vi "Open Motors.vi"() -> ()   [LabVIEW 2018]
uses:
  <vilib>/Rock Robotics/WPI/ThirdParty/Phoenix-LabVIEW/Motor Controller/Controls/CTRE_Phoenix_MotorControl_StatusFrameEnhanced.ctl
  <vilib>/Rock Robotics/WPI/ThirdParty/Phoenix-LabVIEW/Motor Controller/Controls/CTRE_Phoenix_MotorControl_EnhancedMotorControllerConfigurables.ctl
  <vilib>/Rock Robotics/WPI/ThirdParty/Phoenix-LabVIEW/Motor Controller/Controls/CTRE_Phoenix_MotorControl_BaseConfigurables.ctl
  <vilib>/Rock Robotics/WPI/ThirdParty/Phoenix-LabVIEW/Motor Controller/Controls/CTRE_Phoenix_MotorControl_VelocityMeasurementPeriod.ctl
  <vilib>/Rock Robotics/WPI/ThirdParty/Phoenix-LabVIEW/Motor Controller/Controls/CTRE_Phoenix_MotorControl_SlotStructure.ctl
  <vilib>/Rock Robotics/WPI/ThirdParty/Phoenix-LabVIEW/Motor Controller/Controls/CTRE_Phoenix_MotorControl_FilterStruct.ctl
  <vilib>/Rock Robotics/WPI/ThirdParty/Phoenix-LabVIEW/Motor Controller/Controls/CTRE_Phoenix_MotorControl_RemoteSourceType.ctl
  <vilib>/Rock Robotics/WPI/ThirdParty/Phoenix-LabVIEW/Controls/CTRE_Phoenix_CustomParamConfiguration.ctl
  <vilib>/Rock Robotics/WPI/ThirdParty/Phoenix-LabVIEW/Motor Controller/Controls/CTRE_Phoenix_MotorControl_FeedbackDevice.ctl
  <vilib>/Rock Robotics/WPI/ThirdParty/Phoenix-LabVIEW/Motor Controller/Controls/CTRE_Phoenix_MotorControl_SensorTermFeedbackDevice_Enhanced.ctl
  <vilib>/Rock Robotics/WPI/ThirdParty/Phoenix-LabVIEW/Motor Controller/Controls/CTRE_Phoenix_MotorControl_LimitSwitchNormal.ctl
  <vilib>/Rock Robotics/WPI/ThirdParty/Phoenix-LabVIEW/Motor Controller/Controls/CTRE_Phoenix_MotorControl_LimitSwitchSource_Local.ctl
  Robot Global Data.vi
  <vilib>/Rock Robotics/WPI/RobotDrive/WPI_RobotDriveOpen4MotorWithExistingMotors.vi
  <vilib>/Rock Robotics/WPI/ThirdParty/Phoenix-LabVIEW/Motor Controller/Controls/CTRE_Phoenix_MotorControl_ControlMode.ctl
  <vilib>/Rock Robotics/WPI/ThirdParty/Phoenix-LabVIEW/Motor Controller/Controls/CTRE_Phoenix_MotorControl_MotionProfileTrajectoryPoint.ctl
  <vilib>/Rock Robotics/WPI/ThirdParty/Phoenix-LabVIEW/Motor Controller/Closed Loop/Motion Profile/CTRE_Phoenix_MotorControl_BufferedTrajectoryPointStream_WriteAll.vi
panel:
  in  "Tune PIDF Manually?":bool
  in  "Front PIDF Values":cluster{"P":dbl, "I":dbl, "D":dbl, "F":dbl}
  in  "Back PIDF Values":cluster{"P":dbl, "I":dbl, "D":dbl, "F":dbl}
  out "Array":dbl[][](array[numeric])
  # "AFTER YOU HAVE THE \nGAINS YOU WANT, \nR-CLICK > DATA \nOPERATIONS > MAKE\nTHE CURRENT VALUE\nDEFAULT\n\nor just hard-code them"
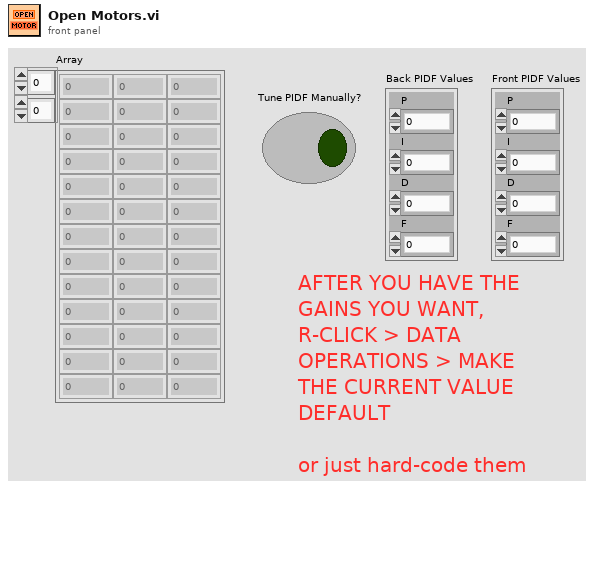
[diagram p1: front panel]
types:
  T1 = typedef "CTRE_Phoenix_MotorControl_EnhancedMotorControllerConfigurables.ctl" = cluster{"Base Configurables":T2, "primaryPID":cluster{"selectedFeedbackCoefficient":dbl, "selectedFeedbackSensor":T8}, "auxiliaryPID":cluster{"selectedFeedbackCoefficient":dbl, "selectedFeedbackSensor":T8}, "sum0Term":T9, "sum1Term":T9, "diff0Term":T9, "diff1Term":T9, "forwardLimitSwitchNormal":T10, "reverseLimitSwitchNormal":T10, "forwardLimitSwitchDeviceID":i32, "reverseLimitSwitchDeviceID":i32, "forwardLimitSwitchSource":T11, "reverseLimitSwitchSource":T11, "peakCurrentLimit":i32, "peakCurrentDuration":i32, "continuousCurrentLimit":i32}
  T2 = typedef "CTRE_Phoenix_MotorControl_BaseConfigurables.ctl" = cluster{"openLoopRamp":dbl, "closedLoopRamp":dbl, "peakOutputForward":dbl, "peakOutputReverse":dbl, "nominalOutputForward":dbl, "nominalOutputReverse":dbl, "neutralDeadband":dbl, "voltageCompSaturation":dbl, "voltageMeasurementFilter":i32, "velocityMeasurementPeriod":T3, "velocityMeasurementWindow":i32, "forwardSoftLimitThreshold":i32, "reverseSoftLimitThreshold":i32, "forwardSoftLimitEnable":bool, "reverseSoftLimitEnable":bool, "slot0":T4, "slot1":T4, "slot2":T4, "slot3":T4, "auxPIDPolarity":bool, "remoteFilter0":T5, "remoteFilter1":T5, "motionCruiseVelocity":i32, "motionAcceleration":i32, "motionProfileTrajectoryPeriod":i32, "feedbackNotContinuous":bool, "remoteSensorClosedLoopDisableNeutralOnLOS":bool, "clearPositionOnLimitF":bool, "clearPositionOnLimitR":bool, "clearPositionOnQuadIdx":bool, "limitSwitchDisableNeutralOnLOS":bool, "softLimitDisableNeutralOnLOS":bool, "pulseWidthPeriod_EdgesPerRot":i32, "pulseWidthPeriod_FilterWindowSz":i32, "customParam":T7, "trajectoryInterpolationEnable":bool}
  T3 = typedef "CTRE_Phoenix_MotorControl_VelocityMeasurementPeriod.ctl" = u16
  T4 = typedef "CTRE_Phoenix_MotorControl_SlotStructure.ctl" = cluster{"P":dbl, "I":dbl, "D":dbl, "F":dbl, "integralZone":dbl, "allowableClosedLoopError":i32, "maxIntegralAccumulator":dbl, "closedLoopPeakOutput":dbl, "closedLoopPeriod":i32}
  T5 = typedef "CTRE_Phoenix_MotorControl_FilterStruct.ctl" = cluster{"remoteSensorDeviceID":u8, "remoteSensorSource":T6}
  T6 = typedef "CTRE_Phoenix_MotorControl_RemoteSourceType.ctl" = enum16{"Off", "Talon SRX Selected Sensor", "Pigeon IMU Yaw", "Pigeon IMU Pitch", "Pigeon IMU Roll", "CANifier Quadrature", "CANifier PWM Input 0", "CANifier PWM Input 1", "CANifier PWM Input 2", "CANifier PWM Input 3", "Gadgeteer Pigeon Yaw", "Gadgeteer Pigeon Pitch", "Gadgeteer Pigeon Roll"}
  T7 = typedef "CTRE_Phoenix_CustomParamConfiguration.ctl" = cluster{"customParam0":i32, "customParam1":i32}
  T8 = typedef "CTRE_Phoenix_MotorControl_FeedbackDevice.ctl" = i8
  T9 = typedef "CTRE_Phoenix_MotorControl_SensorTermFeedbackDevice_Enhanced.ctl" = i8
  T10 = typedef "CTRE_Phoenix_MotorControl_LimitSwitchNormal.ctl" = enum16{"Normally Open", "Normally Closed", "Disabled"}
  T11 = typedef "CTRE_Phoenix_MotorControl_LimitSwitchSource_Local.ctl" = enum16{"Feedback Connector", "Remote Talon SRX", "Remote CANifier", "Deactivated"}
  T12 = typedef "CTRE_Phoenix_MotorControl_StatusFrameEnhanced.ctl" = u16
  T13 = typedef "CTRE_Phoenix_MotorControl_MotionProfileTrajectoryPoint.ctl" = cluster{"Position":dbl, "Velocity":dbl, "Arbitrary Feed Forward":dbl, "Auxiliary Position":dbl, "Auxiliary Velocity":dbl, "Auxiliary Arbitrary Feed Forward":dbl, "Profile Slot Select":i32, "Auxiliary Profile Slot Select":i32, "isLastPoint?":bool, "Zero Position?":bool, "durationMs":u32, "Use Aux PID?":bool}
  T14 = typedef "CTRE_Phoenix_MotorControl_BufferedTrajectoryPointStream_DeviceRef.ctl" = cluster{"Handle":u64, "Library Path":path}
  T15 = typedef "WPI_MotorControlDeviceRef.ctl" = cluster{"DeviceStatus":errorcluster, "Type":T16, "PWM":cluster{"PWM Channel":T17, "DeadBand":T18}, "CAN":cluster{"Device Number":u8, "SetOutput VI Ref":variant, "GetOutput VI Ref":variant, "Enable VI Ref":variant, "Disable VI Ref":variant, "Data":variant}, "Invert":bool, "DIO PWM":cluster{"PWM \"Enable\" Channel":T17, "DIOChannel":T19, "PWM Rate":dbl}}
  T16 = typedef "WPI_MotorControlType.ctl" = enum16{"PWM", "CAN", "DIO PWM"}
  T17 = typedef "FPGA_DIOPWMChannel.ctl" = enum8{"PWM 0", "PWM 1", "PWM 2", "PWM 3", "PWM 4", "PWM 5", "PWM 6", "PWM 7", "PWM 8", "PWM 9", "PWM MXP 0", "PWM MXP 1", "PWM MXP 2", "PWM MXP 3", "PWM MXP 4", "PWM MXP 5", "PWM MXP 6", "PWM MXP 7", "PWM MXP 8", "PWM MXP 9", "Invalid"}
  T18 = typedef "WPI_PWMDeadband.ctl" = cluster{"Name":string, "maxPositivePwm":i32, "minPositivePwm":i32, "centerPwm":i32, "maxNegativePwm":i32, "minNegativePwm":i32, "angularRange":u16}
  T19 = typedef "FPGA_DIOChannel.ctl" = enum8{"DIO 0", "DIO 1", "DIO 2", "DIO 3", "DIO 4", "DIO 5", "DIO 6", "DIO 7", "DIO 8", "DIO 9", "DIO MXP 0", "DIO MXP 1", "DIO MXP 2", "DIO MXP 3", "DIO MXP 4", "DIO MXP 5", "DIO MXP 6", "DIO MXP 7", "DIO MXP 8", "DIO MXP 9", "DIO MXP 10", "DIO MXP 11", "DIO MXP 12", "DIO MXP 13", "DIO MXP 14", "DIO MXP 15", "SPI Port CS1", "SPI Port CS2", "SPI Port CS3", "SPI Port MISO", "SPI Port MOSI", "Invalid"}
  T20 = typedef "Which Robot Enum.ctl" = enum16{"Competition Bot", "Practice Bot", "Code Bot"}
  T21 = typedef "CTRE_Phoenix_MotorControl_ControlMode.ctl" = u16
  T22 = typedef "WPI_RobotDriveDevRef.ctl" = cluster{"DevStatus":errorcluster, "Motors[]":T15[], "Square Inputs":bool, "Max Output":dbl}
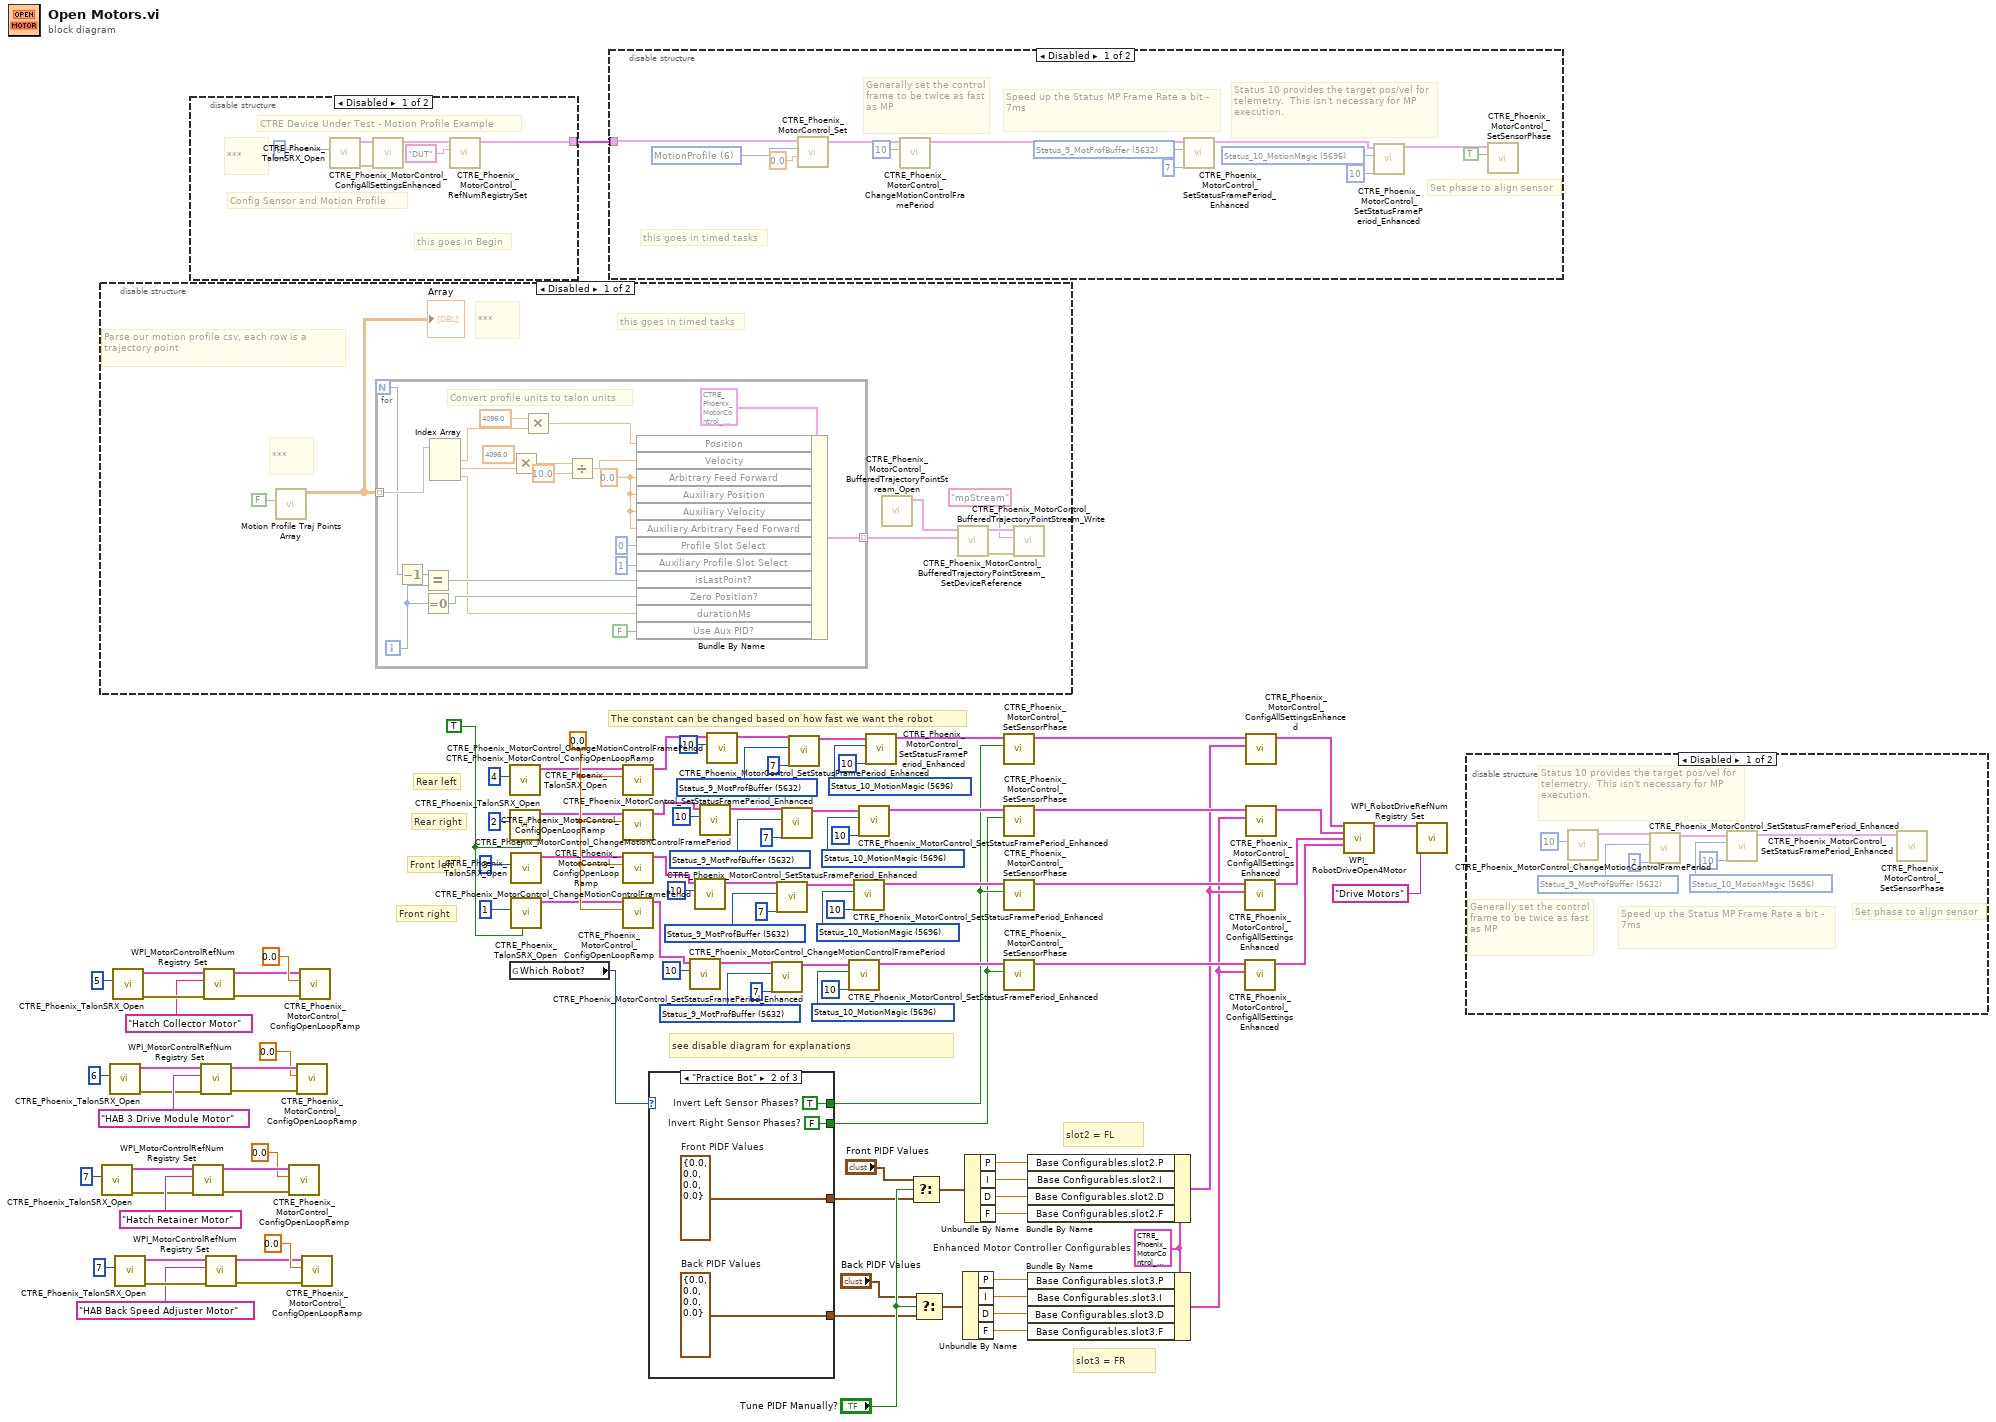
[diagram p0: block diagram]
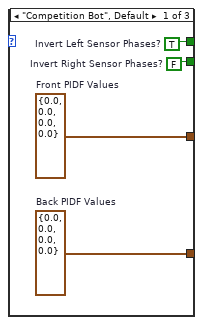
[diagram p3: hidden frame]
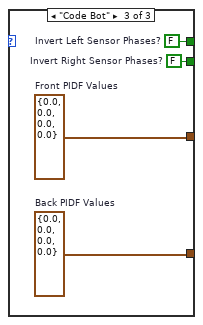
[diagram p4: hidden frame]
diagram:
  w22 = T1 {"Base Configurables"={"openLoopRamp"=0.0, "closedLoopRamp"=0.0, "peakOutputForward"=1.0, "peakOutputReverse"=-1.0, "nominalOutputForward"=0.0, "nominalOutputReverse"=0.0, "neutralDeadband"=0.04, "voltageCompSaturation"=0.0, "voltageMeasurementFilter"=32, "velocityMeasurementPeriod"=100, "velocityMeasurementWindow"=64, "forwardSoftLimitThreshold"=0, "reverseSoftLimitThreshold"=0, "forwardSoftLimitEnable"=FALSE, "reverseSoftLimitEnable"=FALSE, "slot0"={"P"=0.0, "I"=0.0, "D"=0.0, "F"=0.0, "integralZone"=0.0, "allowableClosedLoopError"=0, "maxIntegralAccumulator"=0.0, "closedLoopPeakOutput"=1.0, "closedLoopPeriod"=1}, "slot1"={"P"=0.0, "I"=0.0, "D"=0.0, "F"=0.0, "integralZone"=0.0, "allowableClosedLoopError"=0, "maxIntegralAccumulator"=0.0, "closedLoopPeakOutput"=1.0, "closedLoopPeriod"=1}, "slot2"={"P"=0.0, "I"=0.0, "D"=0.0, "F"=0.0, "integralZone"=0.0, "allowableClosedLoopError"=0, "maxIntegralAccumulator"=0.0, "closedLoopPeakOutput"=1.0, "closedLoopPeriod"=1}, "slot3"={"P"=0.0, "I"=0.0, "D"=0.0, "F"=0.0, "integralZone"=0.0, "allowableClosedLoopError"=0, "maxIntegralAccumulator"=0.0, "closedLoopPeakOutput"=1.0, "closedLoopPeriod"=1}, "auxPIDPolarity"=FALSE, "remoteFilter0"={"remoteSensorDeviceID"=0, "remoteSensorSource"=enum."Off"}, "remoteFilter1"={"remoteSensorDeviceID"=0, "remoteSensorSource"=enum."Off"}, "motionCruiseVelocity"=0, "motionAcceleration"=0, "motionProfileTrajectoryPeriod"=0, "feedbackNotContinuous"=FALSE, "remoteSensorClosedLoopDisableNeutralOnLOS"=FALSE, "clearPositionOnLimitF"=FALSE, "clearPositionOnLimitR"=FALSE, "clearPositionOnQuadIdx"=FALSE, "limitSwitchDisableNeutralOnLOS"=FALSE, "softLimitDisableNeutralOnLOS"=FALSE, "pulseWidthPeriod_EdgesPerRot"=1, "pulseWidthPeriod_FilterWindowSz"=1, "customParam"={"customParam0"=0, "customParam1"=0}, "trajectoryInterpolationEnable"=TRUE}, "primaryPID"={"selectedFeedbackCoefficient"=1.0, "selectedFeedbackSensor"=0}, "auxiliaryPID"={"selectedFeedbackCoefficient"=1.0, "selectedFeedbackSensor"=0}, "sum0Term"=0, "sum1Term"=0, "diff0Term"=0, "diff1Term"=0, "forwardLimitSwitchNormal"=enum."Normally Open", "reverseLimitSwitchNormal"=enum."Normally Open", "forwardLimitSwitchDeviceID"=0, "reverseLimitSwitchDeviceID"=0, "forwardLimitSwitchSource"=enum."Feedback Connector", "reverseLimitSwitchSource"=enum."Feedback Connector", "peakCurrentLimit"=1, "peakCurrentDuration"=1, "continuousCurrentLimit"=1}  # Enhanced Motor Controller Configurables
  w41 = T12 5696 items=["Status_1_General"=5120, "Status_2_Feedback0"=5184, "Status_3_Quadrature"=5248, "Status_4_AinTempVbat"=5312, "Status_6_Misc"=5440, "Status_7_CommStatus"=5504, "Status_8_PulseWidth"=5568, "Status_9_MotProfBuffer"=5632, "Status_10_MotionMagic"=5696, "Status_11_UartGadgeteer"=5760, "Status_12_Feedback1"=5824, "Status_13_Base_PIDF0"=5888, "Status_14_Turn_PIDF1"=5952, "Status_15_FirmwareApiStatus"=6016] ("Status Frame")
  w43 = T12 5632 items=["Status_1_General"=5120, "Status_2_Feedback0"=5184, "Status_3_Quadrature"=5248, "Status_4_AinTempVbat"=5312, "Status_6_Misc"=5440, "Status_7_CommStatus"=5504, "Status_8_PulseWidth"=5568, "Status_9_MotProfBuffer"=5632, "Status_10_MotionMagic"=5696, "Status_11_UartGadgeteer"=5760, "Status_12_Feedback1"=5824, "Status_13_Base_PIDF0"=5888, "Status_14_Turn_PIDF1"=5952, "Status_15_FirmwareApiStatus"=6016] ("Status Frame")
  w49 = T12 5696 items=["Status_1_General"=5120, "Status_2_Feedback0"=5184, "Status_3_Quadrature"=5248, "Status_4_AinTempVbat"=5312, "Status_6_Misc"=5440, "Status_7_CommStatus"=5504, "Status_8_PulseWidth"=5568, "Status_9_MotProfBuffer"=5632, "Status_10_MotionMagic"=5696, "Status_11_UartGadgeteer"=5760, "Status_12_Feedback1"=5824, "Status_13_Base_PIDF0"=5888, "Status_14_Turn_PIDF1"=5952, "Status_15_FirmwareApiStatus"=6016] ("Status Frame")
  w51 = T12 5632 items=["Status_1_General"=5120, "Status_2_Feedback0"=5184, "Status_3_Quadrature"=5248, "Status_4_AinTempVbat"=5312, "Status_6_Misc"=5440, "Status_7_CommStatus"=5504, "Status_8_PulseWidth"=5568, "Status_9_MotProfBuffer"=5632, "Status_10_MotionMagic"=5696, "Status_11_UartGadgeteer"=5760, "Status_12_Feedback1"=5824, "Status_13_Base_PIDF0"=5888, "Status_14_Turn_PIDF1"=5952, "Status_15_FirmwareApiStatus"=6016] ("Status Frame")
  w57 = T12 5696 items=["Status_1_General"=5120, "Status_2_Feedback0"=5184, "Status_3_Quadrature"=5248, "Status_4_AinTempVbat"=5312, "Status_6_Misc"=5440, "Status_7_CommStatus"=5504, "Status_8_PulseWidth"=5568, "Status_9_MotProfBuffer"=5632, "Status_10_MotionMagic"=5696, "Status_11_UartGadgeteer"=5760, "Status_12_Feedback1"=5824, "Status_13_Base_PIDF0"=5888, "Status_14_Turn_PIDF1"=5952, "Status_15_FirmwareApiStatus"=6016] ("Status Frame")
  w59 = T12 5632 items=["Status_1_General"=5120, "Status_2_Feedback0"=5184, "Status_3_Quadrature"=5248, "Status_4_AinTempVbat"=5312, "Status_6_Misc"=5440, "Status_7_CommStatus"=5504, "Status_8_PulseWidth"=5568, "Status_9_MotProfBuffer"=5632, "Status_10_MotionMagic"=5696, "Status_11_UartGadgeteer"=5760, "Status_12_Feedback1"=5824, "Status_13_Base_PIDF0"=5888, "Status_14_Turn_PIDF1"=5952, "Status_15_FirmwareApiStatus"=6016] ("Status Frame")
  w65 = T12 5696 items=["Status_1_General"=5120, "Status_2_Feedback0"=5184, "Status_3_Quadrature"=5248, "Status_4_AinTempVbat"=5312, "Status_6_Misc"=5440, "Status_7_CommStatus"=5504, "Status_8_PulseWidth"=5568, "Status_9_MotProfBuffer"=5632, "Status_10_MotionMagic"=5696, "Status_11_UartGadgeteer"=5760, "Status_12_Feedback1"=5824, "Status_13_Base_PIDF0"=5888, "Status_14_Turn_PIDF1"=5952, "Status_15_FirmwareApiStatus"=6016] ("Status Frame")
  w67 = T12 5632 items=["Status_1_General"=5120, "Status_2_Feedback0"=5184, "Status_3_Quadrature"=5248, "Status_4_AinTempVbat"=5312, "Status_6_Misc"=5440, "Status_7_CommStatus"=5504, "Status_8_PulseWidth"=5568, "Status_9_MotProfBuffer"=5632, "Status_10_MotionMagic"=5696, "Status_11_UartGadgeteer"=5760, "Status_12_Feedback1"=5824, "Status_13_Base_PIDF0"=5888, "Status_14_Turn_PIDF1"=5952, "Status_15_FirmwareApiStatus"=6016] ("Status Frame")
  w90 = TRUE
  w97 = 0.0
  # "slot3 = FR"
  # "slot2 = FL"
  # "see disable diagram for explanations"
  # "Front right"
  # "Front left"
  # "Rear right"
  # "Rear left"
  # "The constant can be changed based on how fast we want the robot"
  n1 = disable-structure shown="Disabled" {
    frame Disabled {
      # "this goes in timed tasks"
      # "***"
      # "***"
      # "Parse our motion profile csv, each row is a trajectory point"
      n2 = call "Motion Profile Traj Points Array.vi"("Read = false, Write = true"=FALSE) -> ("traj. points array out"=w107:dbl[][])  [unwired: 10 in]
      "Array" <- w107
      n3 = for {
        N -> [w127]
        tunnel: w107 -> [w133] mode=indexing
        tunnel: [w123] -> w113 mode=indexing
        i -> [w126]
        w132 = 0.0 ("Arbitrary Feed Forward")
        # "Convert profile units to talon units"
        n4 = Decrement(x=w127) -> (x-1=w128:i32)
        n5 = Equal?(x=w128, y=w126) -> (x = y?=w129:bool)
        n6 = Equal To 0?(x=w126) -> (x = 0?=w125:bool)
        n7 = Index Array(array=w133) -> (element #1=w121:dbl, element #2=w115:dbl, element #3=w122:dbl)  [unwired: 3 in]
        n8 = Multiply(x=4096.0, y=w115) -> (x*y=w117:dbl)
        n9 = Multiply(x=4096.0, y=w121) -> (x*y=w119:dbl)
        n10 = Divide(x=w117, y=10.0) -> (x/y=w114:dbl)
        n11 = Bundle By Name(cluster=T13 {"Position"=0.0, "Velocity"=0.0, "Arbitrary Feed Forward"=0.0, "Auxiliary Position"=0.0, "Auxiliary Velocity"=0.0, "Auxiliary Arbitrary Feed Forward"=0.0, "Profile Slot Select"=0, "Auxiliary Profile Slot Select"=0, "isLastPoint?"=FALSE, "Zero Position?"=FALSE, "durationMs"=0, "Use Aux PID?"=FALSE} ("Trajectory Point"), "Position"=w119, "Velocity"=w114, "Arbitrary Feed Forward"=w132, "Auxiliary Position"=w132, "Auxiliary Velocity"=w132, "Auxiliary Arbitrary Feed Forward"=w132, "Profile Slot Select"=0, "Auxiliary Profile Slot Select"=1, "isLastPoint?"=w129, "Zero Position?"=w125, "durationMs"=w122, "Use Aux PID?"=FALSE) -> (w123:T13)
      }
      n12 = call <vilib>:"CTRE_Phoenix_MotorControl_BufferedTrajectoryPointStream_Open.vi"() -> ("BufferedTrajectoryPointStream_DevRef"=w112:T14)  [unwired: 10 in, 1 out]
      n13 = call-poly <vilib>:"CTRE_Phoenix_MotorControl_BufferedTrajectoryPointStream_Write.vi"("Motion Profile Trajectory Point Array"=w113, "BufferedTrajectoryPointStream_DevRef"=w112) -> ("error out"=w110:errorcluster, "BufferedTrajectoryPointStream_DevRef"=w111:T14)  [unwired: 8 in]
      n14 = call <vilib>:"CTRE_Phoenix_MotorControl_BufferedTrajectoryPointStream_SetDeviceReference.vi"("error in (no error)"=w110, "refnum name"="mpStream", "BufferedTrajectoryPointStream_DevRef"=w111) -> ()  [unwired: 7 in, 2 out]
    }
    frame Enabled {
    }
  }
  n15 = call <vilib>:"CTRE_Phoenix_TalonSRX_Open.vi"("Device Number"=u8 7) -> ("error out"=w75:errorcluster, "CAN Talon SRX Ref"=w78:T15)  [unwired: 9 in]
  n16 = call <vilib>:"CTRE_Phoenix_TalonSRX_Open.vi"("Device Number"=u8 6) -> ("error out"=w85:errorcluster, "CAN Talon SRX Ref"=w88:T15)  [unwired: 9 in]
  n17 = call <vilib>:"CTRE_Phoenix_TalonSRX_Open.vi"("Device Number"=u8 5) -> ("error out"=w104:errorcluster, "CAN Talon SRX Ref"=w101:T15)  [unwired: 9 in]
  n18 = call <vilib>:"CTRE_Phoenix_TalonSRX_Open.vi"("Device Number"=u8 7) -> ("error out"=w5:errorcluster, "CAN Talon SRX Ref"=w2:T15)  [unwired: 9 in]
  n19 = disable-structure shown="Disabled" {
    disable-tunnel: [w139 _] -> w80
    frame Disabled {
      # "this goes in Begin"
      # "***"
      # "Config Sensor and Motion Profile"
      # "CTRE Device Under Test - Motion Profile Example"
      n20 = call <vilib>:"CTRE_Phoenix_TalonSRX_Open.vi"("Device Number"=u8 6) -> ("error out"=w138:errorcluster, "CAN Talon SRX Ref"=w137:T15)  [unwired: 9 in]
      n21 = call <vilib>:"CTRE_Phoenix_MotorControl_ConfigAllSettingsEnhanced.vi"("error in (no error)"=w138, "PhoenixMotorControlDevRef"=w137) -> ("PhoenixMotorControlDevRef"=w136:T15, "Enhanced Motor Controller Configurables"=w135:T1)  [unwired: 7 in, 1 out]
      n22 = call <vilib>:"CTRE_Phoenix_MotorControl_RefNumRegistrySet.vi"("refnum name"="DUT", "PhoenixMotorControlDevRef"=w136) -> ("PhoenixMotorControlDevRef"=w139:T15)  [unwired: 8 in, 1 out]
    }
    frame Enabled {
    }
  }
  n23 = call <vilib>:"WPI_MotorControlRefNum Registry Set.vi"("error in (no error)"=w75, "refnum name"="Hatch Retainer Motor", "MotorControlDevRef"=w78) -> ("error out"=w74:errorcluster, "MotorControlDevRef"=w76:T15)  [unwired: 7 in]
  n24 = call <vilib>:"WPI_MotorControlRefNum Registry Set.vi"("error in (no error)"=w85, "refnum name"="HAB 3 Drive Module Motor", "MotorControlDevRef"=w88) -> ("error out"=w84:errorcluster, "MotorControlDevRef"=w86:T15)  [unwired: 7 in]
  n25 = call <vilib>:"WPI_MotorControlRefNum Registry Set.vi"("error in (no error)"=w104, "refnum name"="Hatch Collector Motor", "MotorControlDevRef"=w101) -> ("error out"=w105:errorcluster, "MotorControlDevRef"=w103:T15)  [unwired: 7 in]
  n26 = call <vilib>:"WPI_MotorControlRefNum Registry Set.vi"("error in (no error)"=w5, "refnum name"="HAB Back Speed Adjuster Motor", "MotorControlDevRef"=w2) -> ("error out"=w6:errorcluster, "MotorControlDevRef"=w4:T15)  [unwired: 7 in]
  n27 = call <vilib>:"CTRE_Phoenix_MotorControl_ConfigOpenLoopRamp.vi"("error in (no error)"=w74, "secondsFromNeutralToFull"=0.0, "PhoenixMotorControlDevRef"=w76) -> ()  [unwired: 7 in, 2 out]
  n28 = call <vilib>:"CTRE_Phoenix_MotorControl_ConfigOpenLoopRamp.vi"("error in (no error)"=w84, "secondsFromNeutralToFull"=0.0, "PhoenixMotorControlDevRef"=w86) -> ()  [unwired: 7 in, 2 out]
  n29 = call <vilib>:"CTRE_Phoenix_MotorControl_ConfigOpenLoopRamp.vi"("error in (no error)"=w105, "secondsFromNeutralToFull"=0.0, "PhoenixMotorControlDevRef"=w103) -> ()  [unwired: 7 in, 2 out]
  n30 = call <vilib>:"CTRE_Phoenix_MotorControl_ConfigOpenLoopRamp.vi"("error in (no error)"=w6, "secondsFromNeutralToFull"=0.0, "PhoenixMotorControlDevRef"=w4) -> ()  [unwired: 7 in, 2 out]
  n31 = call <vilib>:"CTRE_Phoenix_TalonSRX_Open.vi"("Device Number"=u8 4) -> ("CAN Talon SRX Ref"=w92:T15)  [unwired: 9 in, 1 out]
  n32 = call <vilib>:"CTRE_Phoenix_TalonSRX_Open.vi"("Invert"=w90, "Device Number"=u8 2) -> ("CAN Talon SRX Ref"=w93:T15)  [unwired: 8 in, 1 out]
  n33 = global read "Robot Global Data.vi" "Which Robot?"() -> (w72:T20)
  n34 = call <vilib>:"CTRE_Phoenix_TalonSRX_Open.vi"("Device Number"=u8 3) -> ("CAN Talon SRX Ref"=w96:T15)  [unwired: 9 in, 1 out]
  n35 = call <vilib>:"CTRE_Phoenix_TalonSRX_Open.vi"("Invert"=w90, "Device Number"=u8 1) -> ("CAN Talon SRX Ref"=w95:T15)  [unwired: 8 in, 1 out]
  n36 = disable-structure shown="Disabled" {
    disable-tunnel: w80 -> [w152 _]
    frame Disabled {
      w149 = T12 5696 items=["Status_1_General"=5120, "Status_2_Feedback0"=5184, "Status_3_Quadrature"=5248, "Status_4_AinTempVbat"=5312, "Status_6_Misc"=5440, "Status_7_CommStatus"=5504, "Status_8_PulseWidth"=5568, "Status_9_MotProfBuffer"=5632, "Status_10_MotionMagic"=5696, "Status_11_UartGadgeteer"=5760, "Status_12_Feedback1"=5824, "Status_13_Base_PIDF0"=5888, "Status_14_Turn_PIDF1"=5952, "Status_15_FirmwareApiStatus"=6016] ("Status Frame")
      w151 = T12 5632 items=["Status_1_General"=5120, "Status_2_Feedback0"=5184, "Status_3_Quadrature"=5248, "Status_4_AinTempVbat"=5312, "Status_6_Misc"=5440, "Status_7_CommStatus"=5504, "Status_8_PulseWidth"=5568, "Status_9_MotProfBuffer"=5632, "Status_10_MotionMagic"=5696, "Status_11_UartGadgeteer"=5760, "Status_12_Feedback1"=5824, "Status_13_Base_PIDF0"=5888, "Status_14_Turn_PIDF1"=5952, "Status_15_FirmwareApiStatus"=6016] ("Status Frame")
      w154 = T21 6 items=["PercentOutput"=0, "Position"=1, "Velocity"=2, "Current"=3, "Follower"=5, "MotionProfile"=6, "MotionMagic"=7, "MotionMagicArc"=8, "MotionProfileArc"=10, "Disabled"=15] ("Control Mode")
      # "this goes in timed tasks"
      # "Set phase to align sensor"
      # "Generally set the control frame to be twice as fast as MP"
      # "Status 10 provides the target pos/vel for telemetry.  This isn't necessary for MP execution."
      # "Speed up the Status MP Frame Rate a bit - 7ms"
      n37 = call <vilib>:"CTRE_Phoenix_MotorControl_Set.vi"("Output"=0.0, "Control Mode"=w154, "PhoenixMotorControlDevRef"=w152) -> ("PhoenixMotorControlDevRef"=w144:T15)  [unwired: 7 in, 1 out]
      n38 = call <vilib>:"CTRE_Phoenix_MotorControl_ChangeMotionControlFramePeriod.vi"("periodMs"=10, "PhoenixMotorControlDevRef"=w144) -> ("PhoenixMotorControlDevRef"=w146:T15)  [unwired: 8 in, 1 out]
      n39 = call <vilib>:"CTRE_Phoenix_MotorControl_SetStatusFramePeriod_Enhanced.vi"("periodMs"=7, "Status Frame"=w151, "PhoenixMotorControlDevRef"=w146) -> ("PhoenixMotorControlDevRef"=w147:T15)  [unwired: 7 in, 1 out]
      n40 = call <vilib>:"CTRE_Phoenix_MotorControl_SetStatusFramePeriod_Enhanced.vi"("periodMs"=10, "Status Frame"=w149, "PhoenixMotorControlDevRef"=w147) -> ("PhoenixMotorControlDevRef"=w142:T15)  [unwired: 7 in, 1 out]
      n41 = call <vilib>:"CTRE_Phoenix_MotorControl_SetSensorPhase.vi"("PhaseSensor"=TRUE, "PhoenixMotorControlDevRef"=w142) -> ()  [unwired: 8 in, 2 out]
    }
    frame Enabled {
    }
  }
  n42 = call <vilib>:"CTRE_Phoenix_MotorControl_ConfigOpenLoopRamp.vi"("secondsFromNeutralToFull"=w97, "PhoenixMotorControlDevRef"=w92) -> ("PhoenixMotorControlDevRef"=w39:T15)  [unwired: 8 in, 1 out]
  n43 = call <vilib>:"CTRE_Phoenix_MotorControl_ConfigOpenLoopRamp.vi"("secondsFromNeutralToFull"=w97, "PhoenixMotorControlDevRef"=w93) -> ("PhoenixMotorControlDevRef"=w38:T15)  [unwired: 8 in, 1 out]
  n44 = call <vilib>:"CTRE_Phoenix_MotorControl_ConfigOpenLoopRamp.vi"("secondsFromNeutralToFull"=w97, "PhoenixMotorControlDevRef"=w96) -> ("PhoenixMotorControlDevRef"=w37:T15)  [unwired: 8 in, 1 out]
  n45 = call <vilib>:"CTRE_Phoenix_MotorControl_ConfigOpenLoopRamp.vi"("secondsFromNeutralToFull"=w97, "PhoenixMotorControlDevRef"=w95) -> ("PhoenixMotorControlDevRef"=w36:T15)  [unwired: 8 in, 1 out]
  n46 = case shown="\"Practice Bot\"" w72 {
    tunnel: [w158 w162 w166] -> w31
    tunnel: [w157 w161 w165] -> w30
    tunnel: [w156 w160 w164] -> w27
    tunnel: [w155 w159 w163] -> w28
    frame "Competition Bot", Default {
      w155 = cluster{"P":dbl, " I":dbl, "D":dbl, "F":dbl} {"P"=0.0, " I"=0.0, "D"=0.0, "F"=0.0}  # Back PIDF Values
      w156 = cluster{"P":dbl, " I":dbl, "D":dbl, "F":dbl} {"P"=0.0, " I"=0.0, "D"=0.0, "F"=0.0}  # Front PIDF Values
      w157 = FALSE  # Invert Right Sensor Phases?
      w158 = TRUE  # Invert Left Sensor Phases?
    }
    frame "Practice Bot" {
      w159 = cluster{"P":dbl, " I":dbl, "D":dbl, "F":dbl} {"P"=0.0, " I"=0.0, "D"=0.0, "F"=0.0}  # Back PIDF Values
      w160 = cluster{"P":dbl, " I":dbl, "D":dbl, "F":dbl} {"P"=0.0, " I"=0.0, "D"=0.0, "F"=0.0}  # Front PIDF Values
      w161 = FALSE  # Invert Right Sensor Phases?
      w162 = TRUE  # Invert Left Sensor Phases?
    }
    frame "Code Bot" {
      w163 = cluster{"P":dbl, " I":dbl, "D":dbl, "F":dbl} {"P"=0.0, " I"=0.0, "D"=0.0, "F"=0.0}  # Back PIDF Values
      w164 = cluster{"P":dbl, " I":dbl, "D":dbl, "F":dbl} {"P"=0.0, " I"=0.0, "D"=0.0, "F"=0.0}  # Front PIDF Values
      w165 = FALSE  # Invert Right Sensor Phases?
      w166 = FALSE  # Invert Left Sensor Phases?
    }
  }
  n47 = call <vilib>:"CTRE_Phoenix_MotorControl_ChangeMotionControlFramePeriod.vi"("periodMs"=10, "PhoenixMotorControlDevRef"=w36) -> ("PhoenixMotorControlDevRef"=w44:T15)  [unwired: 8 in, 1 out]
  n48 = call <vilib>:"CTRE_Phoenix_MotorControl_ChangeMotionControlFramePeriod.vi"("periodMs"=10, "PhoenixMotorControlDevRef"=w37) -> ("PhoenixMotorControlDevRef"=w52:T15)  [unwired: 8 in, 1 out]
  n49 = call <vilib>:"CTRE_Phoenix_MotorControl_ChangeMotionControlFramePeriod.vi"("periodMs"=10, "PhoenixMotorControlDevRef"=w38) -> ("PhoenixMotorControlDevRef"=w60:T15)  [unwired: 8 in, 1 out]
  n50 = call <vilib>:"CTRE_Phoenix_MotorControl_ChangeMotionControlFramePeriod.vi"("periodMs"=10, "PhoenixMotorControlDevRef"=w39) -> ("PhoenixMotorControlDevRef"=w68:T15)  [unwired: 8 in, 1 out]
  n51 = call <vilib>:"CTRE_Phoenix_MotorControl_SetStatusFramePeriod_Enhanced.vi"("periodMs"=7, "Status Frame"=w43, "PhoenixMotorControlDevRef"=w44) -> ("PhoenixMotorControlDevRef"=w46:T15)  [unwired: 7 in, 1 out]
  n52 = call <vilib>:"CTRE_Phoenix_MotorControl_SetStatusFramePeriod_Enhanced.vi"("periodMs"=7, "Status Frame"=w51, "PhoenixMotorControlDevRef"=w52) -> ("PhoenixMotorControlDevRef"=w54:T15)  [unwired: 7 in, 1 out]
  n53 = call <vilib>:"CTRE_Phoenix_MotorControl_SetStatusFramePeriod_Enhanced.vi"("periodMs"=7, "Status Frame"=w59, "PhoenixMotorControlDevRef"=w60) -> ("PhoenixMotorControlDevRef"=w62:T15)  [unwired: 7 in, 1 out]
  n54 = call <vilib>:"CTRE_Phoenix_MotorControl_SetStatusFramePeriod_Enhanced.vi"("periodMs"=7, "Status Frame"=w67, "PhoenixMotorControlDevRef"=w68) -> ("PhoenixMotorControlDevRef"=w70:T15)  [unwired: 7 in, 1 out]
  n55 = call <vilib>:"CTRE_Phoenix_MotorControl_SetStatusFramePeriod_Enhanced.vi"("periodMs"=10, "Status Frame"=w41, "PhoenixMotorControlDevRef"=w46) -> ("PhoenixMotorControlDevRef"=w47:T15)  [unwired: 7 in, 1 out]
  n56 = call <vilib>:"CTRE_Phoenix_MotorControl_SetStatusFramePeriod_Enhanced.vi"("periodMs"=10, "Status Frame"=w49, "PhoenixMotorControlDevRef"=w54) -> ("PhoenixMotorControlDevRef"=w55:T15)  [unwired: 7 in, 1 out]
  n57 = call <vilib>:"CTRE_Phoenix_MotorControl_SetStatusFramePeriod_Enhanced.vi"("periodMs"=10, "Status Frame"=w57, "PhoenixMotorControlDevRef"=w62) -> ("PhoenixMotorControlDevRef"=w63:T15)  [unwired: 7 in, 1 out]
  n58 = call <vilib>:"CTRE_Phoenix_MotorControl_SetStatusFramePeriod_Enhanced.vi"("periodMs"=10, "Status Frame"=w65, "PhoenixMotorControlDevRef"=w70) -> ("PhoenixMotorControlDevRef"=w71:T15)  [unwired: 7 in, 1 out]
  n59 = Select(t="Front PIDF Values", s="Tune PIDF Manually?", f=w27) -> (s? t:f=w24:cluster{"P":dbl, " I":dbl, "D":dbl, "F":dbl})
  n60 = Select(t="Back PIDF Values", s="Tune PIDF Manually?", f=w28) -> (s? t:f=w23:cluster{"P":dbl, " I":dbl, "D":dbl, "F":dbl})
  n61 = Unbundle By Name(w23) -> ("P"=w17:dbl, "I"=w16:dbl, "D"=w15:dbl, "F"=w14:dbl)
  n62 = Unbundle By Name(w24) -> ("P"=w21:dbl, "I"=w20:dbl, "D"=w19:dbl, "F"=w18:dbl)
  n63 = call <vilib>:"CTRE_Phoenix_MotorControl_SetSensorPhase.vi"("PhaseSensor"=w31, "PhoenixMotorControlDevRef"=w71) -> ("PhoenixMotorControlDevRef"=w34:T15)  [unwired: 8 in, 1 out]
  n64 = call <vilib>:"CTRE_Phoenix_MotorControl_SetSensorPhase.vi"("PhaseSensor"=w30, "PhoenixMotorControlDevRef"=w63) -> ("PhoenixMotorControlDevRef"=w33:T15)  [unwired: 8 in, 1 out]
  n65 = call <vilib>:"CTRE_Phoenix_MotorControl_SetSensorPhase.vi"("PhaseSensor"=w31, "PhoenixMotorControlDevRef"=w55) -> ("PhoenixMotorControlDevRef"=w32:T15)  [unwired: 8 in, 1 out]
  n66 = call <vilib>:"CTRE_Phoenix_MotorControl_SetSensorPhase.vi"("PhaseSensor"=w30, "PhoenixMotorControlDevRef"=w47) -> ("PhoenixMotorControlDevRef"=w35:T15)  [unwired: 8 in, 1 out]
  n67 = Bundle By Name(cluster=w22, "Base Configurables.slot2.P"=w21, "Base Configurables.slot2.I"=w20, "Base Configurables.slot2.D"=w19, "Base Configurables.slot2.F"=w18) -> (w9:T1)
  n68 = Bundle By Name(cluster=w22, "Base Configurables.slot3.P"=w17, "Base Configurables.slot3.I"=w16, "Base Configurables.slot3.D"=w15, "Base Configurables.slot3.F"=w14) -> (w8:T1)
  n69 = call <vilib>:"CTRE_Phoenix_MotorControl_ConfigAllSettingsEnhanced.vi"("Enhanced Motor Controller Configurables"=w9, "PhoenixMotorControlDevRef"=w32) -> ("PhoenixMotorControlDevRef"=w11:T15)  [unwired: 8 in, 1 out]
  n70 = call <vilib>:"CTRE_Phoenix_MotorControl_ConfigAllSettingsEnhanced.vi"("Enhanced Motor Controller Configurables"=w8, "PhoenixMotorControlDevRef"=w35) -> ("PhoenixMotorControlDevRef"=w10:T15)  [unwired: 8 in, 1 out]
  n71 = call <vilib>:"CTRE_Phoenix_MotorControl_ConfigAllSettingsEnhanced.vi"("Enhanced Motor Controller Configurables"=w9, "PhoenixMotorControlDevRef"=w34) -> ("PhoenixMotorControlDevRef"=w13:T15)  [unwired: 8 in, 1 out]
  n72 = call <vilib>:"CTRE_Phoenix_MotorControl_ConfigAllSettingsEnhanced.vi"("Enhanced Motor Controller Configurables"=w8, "PhoenixMotorControlDevRef"=w33) -> ("PhoenixMotorControlDevRef"=w12:T15)  [unwired: 8 in, 1 out]
  n73 = call-poly <vilib>:"WPI_RobotDriveOpen4Motor.vi"("Rear Left Motor Dev Ref"=w13, "Rear Right Motor Dev Ref"=w12, "Front Left Motor Dev Ref"=w11, "Front Right Motor Dev Ref"=w10) -> ("RobotDriveDevRef"=w98:T22)  [unwired: 10 in, 1 out]
  n74 = call <vilib>:"WPI_RobotDriveRefNum Registry Set.vi"("refnum name"="Drive Motors", "RobotDriveDevRef"=w98) -> ()  [unwired: 8 in, 2 out]
  n75 = disable-structure shown="Disabled" {
    frame Disabled {
      w168 = T12 5696 items=["Status_1_General"=5120, "Status_2_Feedback0"=5184, "Status_3_Quadrature"=5248, "Status_4_AinTempVbat"=5312, "Status_6_Misc"=5440, "Status_7_CommStatus"=5504, "Status_8_PulseWidth"=5568, "Status_9_MotProfBuffer"=5632, "Status_10_MotionMagic"=5696, "Status_11_UartGadgeteer"=5760, "Status_12_Feedback1"=5824, "Status_13_Base_PIDF0"=5888, "Status_14_Turn_PIDF1"=5952, "Status_15_FirmwareApiStatus"=6016] ("Status Frame")
      w170 = T12 5632 items=["Status_1_General"=5120, "Status_2_Feedback0"=5184, "Status_3_Quadrature"=5248, "Status_4_AinTempVbat"=5312, "Status_6_Misc"=5440, "Status_7_CommStatus"=5504, "Status_8_PulseWidth"=5568, "Status_9_MotProfBuffer"=5632, "Status_10_MotionMagic"=5696, "Status_11_UartGadgeteer"=5760, "Status_12_Feedback1"=5824, "Status_13_Base_PIDF0"=5888, "Status_14_Turn_PIDF1"=5952, "Status_15_FirmwareApiStatus"=6016] ("Status Frame")
      # "Set phase to align sensor"
      # "Generally set the control frame to be twice as fast as MP"
      # "Status 10 provides the target pos/vel for telemetry.  This isn't necessary for MP execution."
      # "Speed up the Status MP Frame Rate a bit - 7ms"
      n76 = call <vilib>:"CTRE_Phoenix_MotorControl_ChangeMotionControlFramePeriod.vi"("periodMs"=10) -> ("PhoenixMotorControlDevRef"=w171:T15)  [unwired: 9 in, 1 out]
      n77 = call <vilib>:"CTRE_Phoenix_MotorControl_SetStatusFramePeriod_Enhanced.vi"("periodMs"=7, "Status Frame"=w170, "PhoenixMotorControlDevRef"=w171) -> ("PhoenixMotorControlDevRef"=w173:T15)  [unwired: 7 in, 1 out]
      n78 = call <vilib>:"CTRE_Phoenix_MotorControl_SetStatusFramePeriod_Enhanced.vi"("periodMs"=10, "Status Frame"=w168, "PhoenixMotorControlDevRef"=w173) -> ("PhoenixMotorControlDevRef"=w174:T15)  [unwired: 7 in, 1 out]
      n79 = call <vilib>:"CTRE_Phoenix_MotorControl_SetSensorPhase.vi"("PhoenixMotorControlDevRef"=w174) -> ()  [unwired: 9 in, 2 out]
    }
    frame Enabled {
    }
  }
